vi "INTELLIFAUCET Temp-Flow.vi"(6 "Debug":bool, 8 "Error In":errorcluster, 10 "TEMP,FLOW":T1, 11 "VISA session":refnum<visa-resource-name>="MW100") -> (0 "Error Out":errorcluster, 3 "dup VISA session":refnum<visa-resource-name>)   [LabVIEW 2023]
uses:
  MW100/Type Definitions/HEWH MW100 Channel Numbers.ctl
  Type Definitions/HEWH Normally Open Valve Control.ctl
  Type Definitions/INTELLIFAUCT Temp Flow.ctl
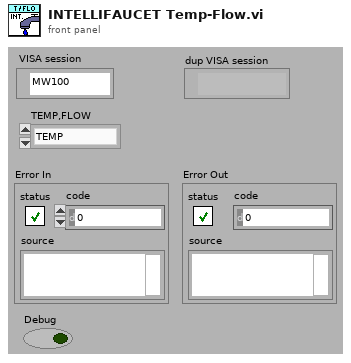
[diagram p1: front panel]
types:
  T1 = typedef "INTELLIFAUCT Temp Flow.ctl" = enum8{"TEMP", "FLOW", "Prop Valve"}
  T2 = typedef "HEWH MW100 Channel Numbers.ctl" = string
  T3 = typedef "HEWH Normally Open Valve Control.ctl" = string
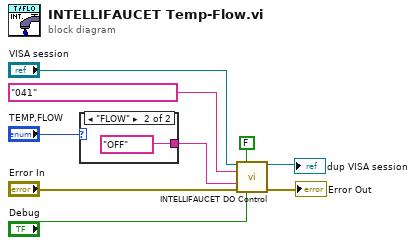
[diagram p0: block diagram]
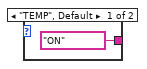
[diagram p2: hidden frame]
diagram:
  n1 = case shown="\"FLOW\"" "TEMP,FLOW" {
    tunnel: [T3 "ON" ("Normally Open Valve") T3 "OFF" ("Normally Open Valve")] -> w2
    frame "TEMP", Default {
    }
    frame "FLOW" {
    }
  }
  n2 = call "INTELLIFAUCET DO Control.vi"("VISA session"="VISA session", 1:FALSE ("Normally Closed Valve?"), "HEWH MW100 Channel Numbers"=T2 "041", 9:w2, "Error In"="Error In", 12:"Debug") -> ("dup VISA session"=→"dup VISA session":refnum<visa-resource-name>, "error out"=→"Error Out":errorcluster)  [unwired: 8 in]
